vi "Item Names.vi"() -> ()   [LabVIEW 2013, in "CVT editor node.lvclass"]
uses:
  CVT editor node.lvclass
panel:
  in  "Available Tags":string[][](array[string])
  in  "From CVT":string[](array[string])
  in  "To CVT":string[](array[string])
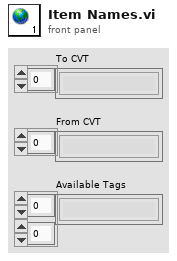
[diagram p1: front panel]
diagram:
